vi "加标回收启动 (子VI).vi"(11 "启动参数":T1(ring)=enum."CODCr") -> (0 "error out":T2={"status"=FALSE, "代码"=4, "source"=""} caption="错误输出" {"代码" items=["执行成功"=1, "执行失败，但不知道原因"=2, "命令请求条件错误"=3, "通讯超时"=4, "系统繁忙不能执行"=5, "系统故障"=6, "没有数据"=100]})   [LabVIEW 2016]
uses:
  PLC/PLC.lvlib
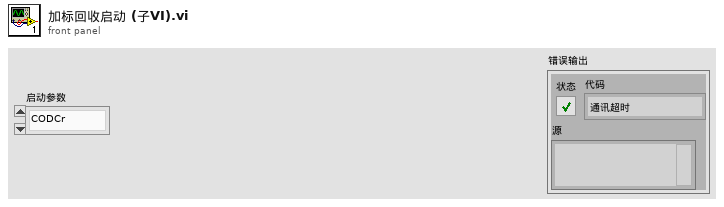
[diagram p1: front panel]
types:
  T1 = enum16{"未选择", "CODMn", "氨氮", "总磷", "总氮", "CODCr"}
  T2 = cluster{"status":bool, "代码":u16, "source":string}
  T3 = enum16{"空闲", "水样测试", "标样核查", "零点核查", "跨度核查", "空白测试", "平行样测试", "质控样", "空白校准", "标样校准", "加标回收"}
  T4 = enum16{"空闲", "水样测试", "标样核查", "零点核查", "跨度核查", "空白测试", "平行样测试", "加标回收", "空白校准", "标样校准", "初始化（清洗）"}
  T5 = cluster{"系统时间":timestamp, "工作状态":u16, "测量模式":enum16{"待机", "连续模式", "周期模式", "定点模式", "受控模式", "手动模式"}, "告警代码":u16, "故障代码":u16, "日志代码":u16, "软件版本":u16, "A":sgl, "B":sgl, "K":sgl, "当前滴定数":sgl, "T":sgl, "H":sgl, "id":u16, "flowid":u16, "量程":u16, "加热实时温度":sgl, "当前ORP值":sgl, "运行时间":sgl, "当前步骤剩余时间":sgl, "结束滴定数":sgl, "注射泵保温温度":sgl}
  T6 = cluster{"R0":i16, "R1":i16, "R2":i16, "R3":i16, "R4":i16, "R5":i16, "R6":i16, "R7":i16, "R8":i16, "R9":i16, "R10":i16, "R11":i16, "R12":i16, "R13":i16, "R14":i16, "R15":i16, "R16":i16, "R17":i16, "R18":i16, "R19":i16, "R20":i16, "R21":i16, "R22":i16, "R23":i16, "R24":i16, "R25":i16, "R26":i16, "R27":i16, "R28":i16, "R29":i16, "R30":i16, "R31":i16, "R32":i16, "R33":i16, "R34":i16, "R35":i16, "R36":i16, "R37":i16, "R38":i16, "R39":i16}
  T7 = enum32{"Bad", "Idle", "Run top level", "Running"}
  T8 = cluster{"系统时间":timestamp, "工作状态":enum16{"空闲", "水样测试", "标样核查", "零点核查", "跨度核查", "空白测试", "平行样测试", "加标回收", "空白校准", "标样校准", "初始化（清洗）"}, "测量模式":enum16{"待机", "连续模式", "周期模式", "定点模式", "受控模式", "手动模式"}, "告警代码":u16, "故障代码":u16, "日志代码":u16, "软件版本":u16, "F0":sgl, "F1":sgl, "F2":sgl, "F3":sgl, "T":sgl, "H":sgl, "id":u16, "flowid":u16, "量程":u16, "总磷控温温度1":sgl, "营养盐控温温度2":sgl, "ADC":sgl}
  T9 = cluster{"系统时间":timestamp, "工作状态":u16, "测量模式":u16, "告警代码":u16, "故障代码":u16, "日志代码":u16, "软件版本":u16, "F0":sgl, "F1":sgl, "F2":sgl, "F3":sgl, "T":sgl, "H":sgl, "id":u16, "flowid":u16, "量程":u16}
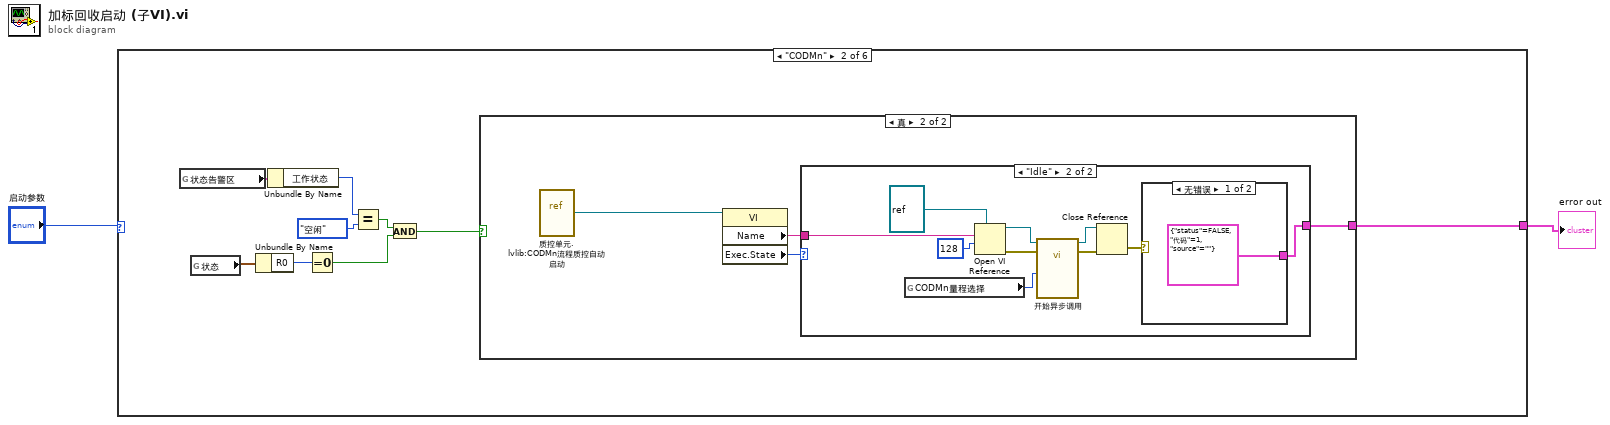
[diagram p0: block diagram]
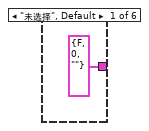
[diagram p2: hidden frame]
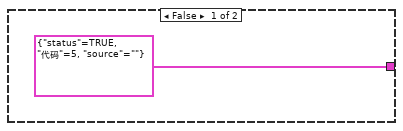
[diagram p3: hidden frame]
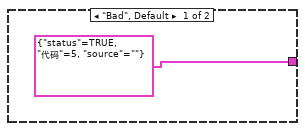
[diagram p4: hidden frame]
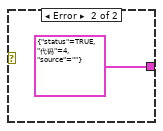
[diagram p5: hidden frame]
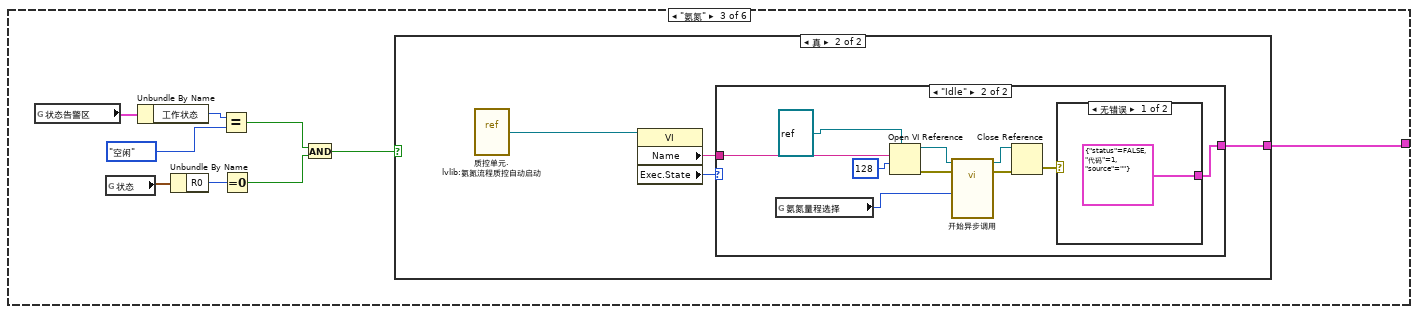
[diagram p6: hidden frame]
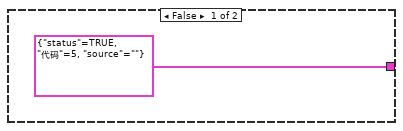
[diagram p7: hidden frame]
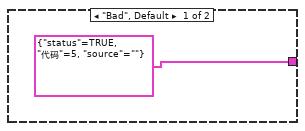
[diagram p8: hidden frame]
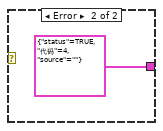
[diagram p9: hidden frame]
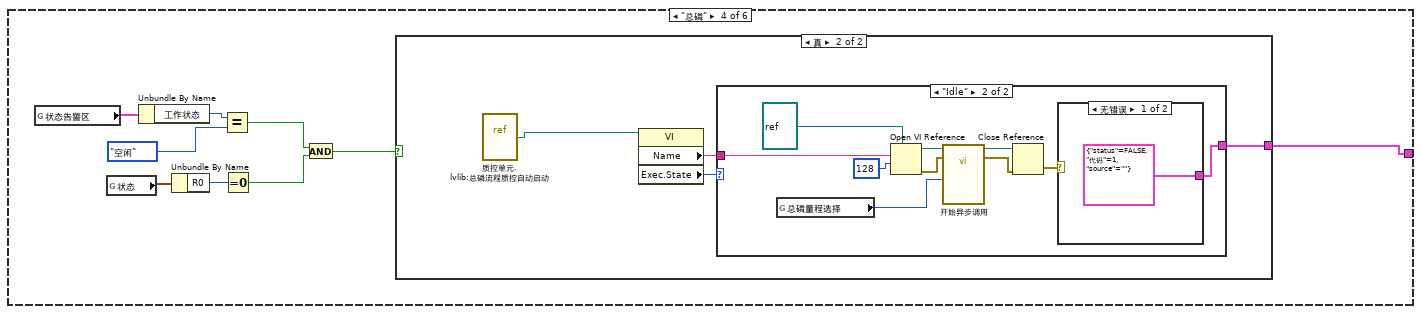
[diagram p10: hidden frame]
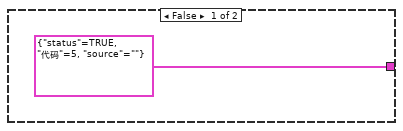
[diagram p11: hidden frame]
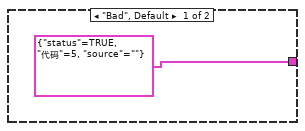
[diagram p12: hidden frame]
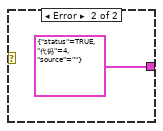
[diagram p13: hidden frame]
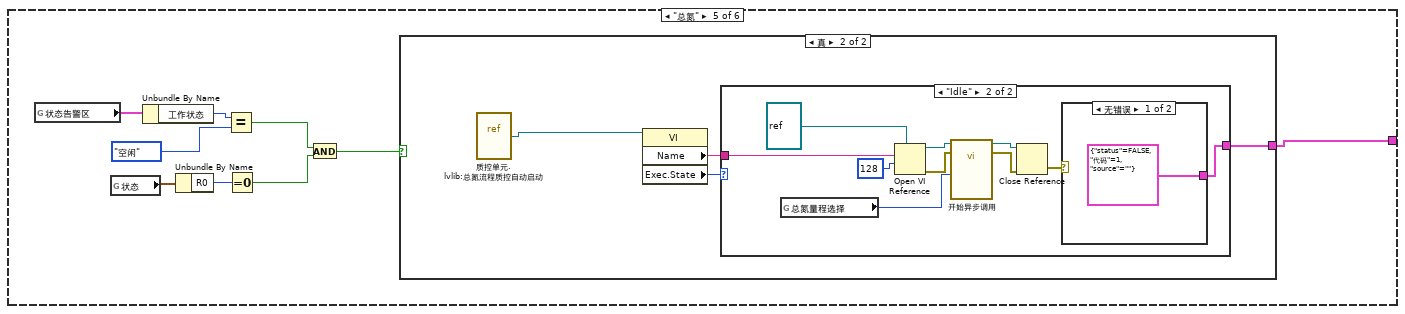
[diagram p14: hidden frame]
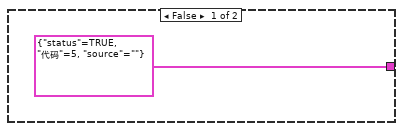
[diagram p15: hidden frame]
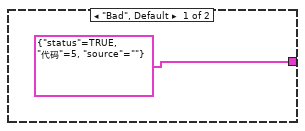
[diagram p16: hidden frame]
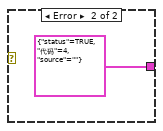
[diagram p17: hidden frame]
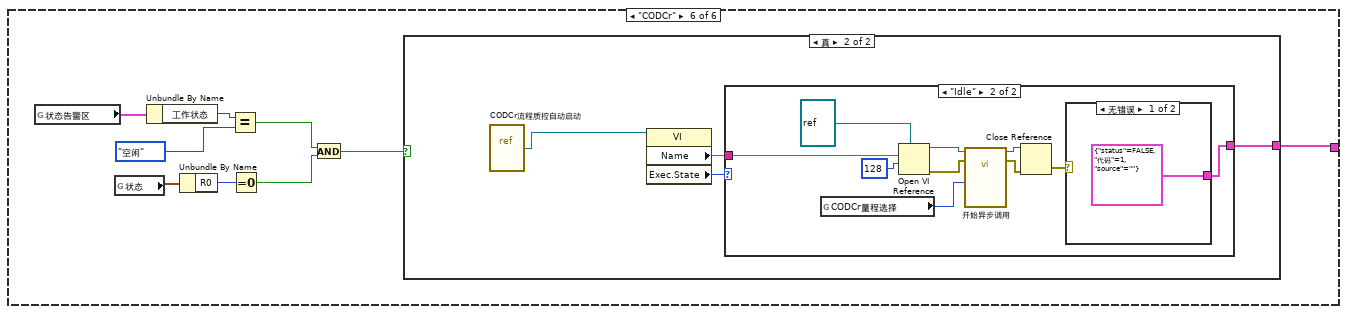
[diagram p18: hidden frame]
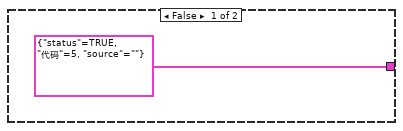
[diagram p19: hidden frame]
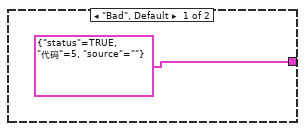
[diagram p20: hidden frame]
diagram:
  n1 = case shown="\"CODMn\"" "启动参数" {
    tunnel: [T2 {"status"=FALSE, "代码"=0, "source"=""} ("error out") w6 w35 w59 w85 w113] -> w1
    frame "未选择", Default {
    }
    frame "CODMn" {
      n2 = global read "VARCODMn全局变量.vi" "状态告警区"() -> (w5:T5)
      n3 = global read "采配水全局变量.vi" "状态"() -> (w10:T6)
      n4 = Unbundle By Name(w10) -> ("R0"=w9:i16)
      n5 = Unbundle By Name(w5) -> ("工作状态"=w4:u16)
      n6 = Equal To 0?(x=w9) -> (x = 0?=w8:bool)
      n7 = Equal?(x=w4, y=T3."空闲") -> (x = y?=w11:bool)
      n8 = And(x=w11, y=w8) -> (x .and. y?=w7:bool)
      n9 = case shown="真" w7 {
        tunnel: [T2 {"status"=TRUE, "代码"=5, "source"=""} ("error out") w14] -> w6
        frame False {
        }
        frame True {
          n10 = vi-ref "质控单元.lvlib:CODMn流程质控自动启动.vi"() -> (w15:refnum<vi>)
          n11 = property class="VI"(reference=w15) -> ("Name"=w17:string, "Exec.State"=w16:T7)  [unwired: 1 in, 2 out]
          n12 = case shown="\"Idle\"" w16 {
            tunnel: w17 -> [_ w25]
            tunnel: [T2 {"status"=TRUE, "代码"=5, "source"=""} ("error out") w21] -> w14
            frame "Bad", Default {
            }
            frame "Idle" {
              n13 = global read "断电保存全局.vi" "CODMn量程选择"() -> (w19:enum32{"H", "L", "AUTO"})
              n14 = Open VI Reference(type specifier VI Refnum (for type only)=refnum<vi> refnum ("类型说明符VI引用句柄（仅用于类型）"), vi path=w25, options=128 ("选项")) -> (vi reference=w20:refnum<vi>, error out=w24:errorcluster)  [unwired: 3 in]
              n15 = call-by-ref "开始异步调用"(reference=w20, error in=w24, "CODMn量程切换"=w19) -> (reference out=w28:refnum<vi>, error out=w23:errorcluster)  [unwired: 10 in]
              n16 = Close Reference(reference=w28, error in (no error)=w23) -> (error out=w22:errorcluster)
              n17 = case shown="无错误" w22 {
                tunnel: [T2 {"status"=FALSE, "代码"=1, "source"=""} ("error out") T2 {"status"=TRUE, "代码"=4, "source"=""} ("error out")] -> w21
                frame No Error {
                }
                frame Error {
                }
              }
            }
          }
        }
      }
    }
    frame "氨氮" {
      n18 = global read "VAR氨氮全局变量.vi" "状态告警区"() -> (w34:T8)
      n19 = global read "采配水全局变量.vi" "状态"() -> (w39:T6)
      n20 = Unbundle By Name(w34) -> ("工作状态"=w33:T4)
      n21 = Unbundle By Name(w39) -> ("R0"=w38:i16)
      n22 = Equal?(x=w33, y=T4."空闲") -> (x = y?=w31:bool)
      n23 = Equal To 0?(x=w38) -> (x = 0?=w37:bool)
      n24 = And(x=w31, y=w37) -> (x .and. y?=w36:bool)
      n25 = case shown="真" w36 {
        tunnel: [T2 {"status"=TRUE, "代码"=5, "source"=""} ("error out") w42] -> w35
        frame False {
        }
        frame True {
          n26 = vi-ref "质控单元.lvlib:氨氮流程质控自动启动.vi"() -> (w41:refnum<vi>)
          n27 = property class="VI"(reference=w41) -> ("Name"=w44:string, "Exec.State"=w43:T7)  [unwired: 1 in, 2 out]
          n28 = case shown="\"Idle\"" w43 {
            tunnel: w44 -> [_ w52]
            tunnel: [T2 {"status"=TRUE, "代码"=5, "source"=""} ("error out") w48] -> w42
            frame "Bad", Default {
            }
            frame "Idle" {
              n29 = global read "断电保存全局.vi" "氨氮量程选择"() -> (w46:enum32{"H", "L", "AUTO"})
              n30 = Open VI Reference(type specifier VI Refnum (for type only)=refnum<vi> refnum ("类型说明符VI引用句柄（仅用于类型）"), vi path=w52, options=128 ("选项")) -> (vi reference=w55:refnum<vi>, error out=w51:errorcluster)  [unwired: 3 in]
              n31 = call-by-ref "开始异步调用"(reference=w55, error in=w51, "氨氮量程切换"=w46) -> (reference out=w54:refnum<vi>, error out=w50:errorcluster)  [unwired: 11 in]
              n32 = Close Reference(reference=w54, error in (no error)=w50) -> (error out=w49:errorcluster)
              n33 = case shown="无错误" w49 {
                tunnel: [T2 {"status"=FALSE, "代码"=1, "source"=""} ("error out") T2 {"status"=TRUE, "代码"=4, "source"=""} ("error out")] -> w48
                frame No Error {
                }
                frame Error {
                }
              }
            }
          }
        }
      }
    }
    frame "总磷" {
      n34 = global read "VAR总磷全局变量.vi" "状态告警区"() -> (w58:T8)
      n35 = global read "采配水全局变量.vi" "状态"() -> (w66:T6)
      n36 = Unbundle By Name(w58) -> ("工作状态"=w62:T4)
      n37 = Unbundle By Name(w66) -> ("R0"=w65:i16)
      n38 = Equal?(x=w62, y=T4."空闲") -> (x = y?=w60:bool)
      n39 = Equal To 0?(x=w65) -> (x = 0?=w64:bool)
      n40 = And(x=w60, y=w64) -> (x .and. y?=w63:bool)
      n41 = case shown="真" w63 {
        tunnel: [T2 {"status"=TRUE, "代码"=5, "source"=""} ("error out") w69] -> w59
        frame False {
        }
        frame True {
          n42 = vi-ref "质控单元.lvlib:总磷流程质控自动启动.vi"() -> (w68:refnum<vi>)
          n43 = property class="VI"(reference=w68) -> ("Name"=w71:string, "Exec.State"=w70:T7)  [unwired: 1 in, 2 out]
          n44 = case shown="\"Idle\"" w70 {
            tunnel: w71 -> [_ w81]
            tunnel: [T2 {"status"=TRUE, "代码"=5, "source"=""} ("error out") w78] -> w69
            frame "Bad", Default {
            }
            frame "Idle" {
              n45 = global read "断电保存全局.vi" "总磷量程选择"() -> (w73:enum32{"H", "L", "AUTO"})
              n46 = Open VI Reference(type specifier VI Refnum (for type only)=refnum<vi> refnum ("类型说明符VI引用句柄（仅用于类型）"), vi path=w81, options=128 ("选项")) -> (vi reference=w76:refnum<vi>, error out=w75:errorcluster)  [unwired: 3 in]
              n47 = call-by-ref "开始异步调用"(reference=w76, error in=w75, "总磷量程切换"=w73) -> (reference out=w74:refnum<vi>, error out=w80:errorcluster)  [unwired: 11 in]
              n48 = Close Reference(reference=w74, error in (no error)=w80) -> (error out=w79:errorcluster)
              n49 = case shown="无错误" w79 {
                tunnel: [T2 {"status"=FALSE, "代码"=1, "source"=""} ("error out") T2 {"status"=TRUE, "代码"=4, "source"=""} ("error out")] -> w78
                frame No Error {
                }
                frame Error {
                }
              }
            }
          }
        }
      }
    }
    frame "总氮" {
      n50 = global read "VAR总氮全局变量.vi" "状态告警区"() -> (w86:T8)
      n51 = global read "采配水全局变量.vi" "状态"() -> (w93:T6)
      n52 = Unbundle By Name(w86) -> ("工作状态"=w89:T4)
      n53 = Unbundle By Name(w93) -> ("R0"=w92:i16)
      n54 = Equal?(x=w89, y=T4."空闲") -> (x = y?=w87:bool)
      n55 = Equal To 0?(x=w92) -> (x = 0?=w91:bool)
      n56 = And(x=w87, y=w91) -> (x .and. y?=w90:bool)
      n57 = case shown="真" w90 {
        tunnel: [T2 {"status"=TRUE, "代码"=5, "source"=""} ("error out") w96] -> w85
        frame False {
        }
        frame True {
          n58 = vi-ref "质控单元.lvlib:总氮流程质控自动启动.vi"() -> (w95:refnum<vi>)
          n59 = property class="VI"(reference=w95) -> ("Name"=w98:string, "Exec.State"=w97:T7)  [unwired: 1 in, 2 out]
          n60 = case shown="\"Idle\"" w97 {
            tunnel: w98 -> [_ w108]
            tunnel: [T2 {"status"=TRUE, "代码"=5, "source"=""} ("error out") w106] -> w96
            frame "Bad", Default {
            }
            frame "Idle" {
              n61 = global read "断电保存全局.vi" "总氮量程选择"() -> (w102:enum32{"H", "L", "AUTO"})
              n62 = Open VI Reference(type specifier VI Refnum (for type only)=refnum<vi> refnum ("类型说明符VI引用句柄（仅用于类型）"), vi path=w108, options=128 ("选项")) -> (vi reference=w104:refnum<vi>, error out=w103:errorcluster)  [unwired: 3 in]
              n63 = call-by-ref "开始异步调用"(reference=w104, error in=w103, "总氮量程切换"=w102) -> (reference out=w101:refnum<vi>, error out=w100:errorcluster)  [unwired: 11 in]
              n64 = Close Reference(reference=w101, error in (no error)=w100) -> (error out=w107:errorcluster)
              n65 = case shown="无错误" w107 {
                tunnel: [T2 {"status"=FALSE, "代码"=1, "source"=""} ("error out") T2 {"status"=TRUE, "代码"=4, "source"=""} ("error out")] -> w106
                frame No Error {
                }
                frame Error {
                }
              }
            }
          }
        }
      }
    }
    frame "CODCr" {
      n66 = global read "CODcr全局变量.vi" "状态告警区"() -> (w112:T9)
      n67 = global read "采配水全局变量.vi" "状态"() -> (w120:T6)
      n68 = Unbundle By Name(w112) -> ("工作状态"=w116:u16)
      n69 = Unbundle By Name(w120) -> ("R0"=w119:i16)
      n70 = Equal?(x=w116, y=T4."空闲") -> (x = y?=w114:bool)
      n71 = Equal To 0?(x=w119) -> (x = 0?=w118:bool)
      n72 = And(x=w114, y=w118) -> (x .and. y?=w117:bool)
      n73 = case shown="真" w117 {
        tunnel: [T2 {"status"=TRUE, "代码"=5, "source"=""} ("error out") w123] -> w113
        frame False {
        }
        frame True {
          n74 = vi-ref "CODCr流程质控自动启动.vi"() -> (w122:refnum<vi>)
          n75 = property class="VI"(reference=w122) -> ("Name"=w125:string, "Exec.State"=w124:T7)  [unwired: 1 in, 2 out]
          n76 = case shown="\"Idle\"" w124 {
            tunnel: w125 -> [_ w135]
            tunnel: [T2 {"status"=TRUE, "代码"=5, "source"=""} ("error out") w133] -> w123
            frame "Bad", Default {
            }
            frame "Idle" {
              n77 = global read "断电保存全局.vi" "CODCr量程选择"() -> (w130:enum32{"H", "L", "AUTO"})
              n78 = Open VI Reference(type specifier VI Refnum (for type only)=refnum<vi> refnum ("类型说明符VI引用句柄（仅用于类型）"), vi path=w135, options=128 ("选项")) -> (vi reference=w131:refnum<vi>, error out=w129:errorcluster)  [unwired: 3 in]
              n79 = call-by-ref "开始异步调用"(reference=w131, error in=w129, "CODCr量程切换"=w130) -> (reference out=w128:refnum<vi>, error out=w127:errorcluster)  [unwired: 10 in]
              n80 = Close Reference(reference=w128, error in (no error)=w127) -> (error out=w134:errorcluster)
              n81 = case shown="无错误" w134 {
                tunnel: [T2 {"status"=FALSE, "代码"=1, "source"=""} ("error out") T2 {"status"=TRUE, "代码"=4, "source"=""} ("error out")] -> w133
                frame No Error {
                }
                frame Error {
                }
              }
            }
          }
        }
      }
    }
  }
  "error out" <- w1
